vi "CalibrateSensors.vi"(5 "Static Load Cell":dbl) -> (1 "Static Load Cell Offset":string)   [LabVIEW 2018]
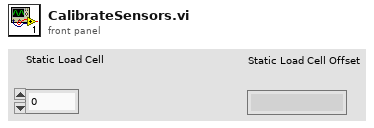
[diagram p1: front panel]
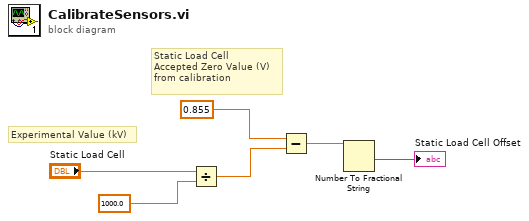
[diagram p0: block diagram]
diagram:
  # "Experimental Value (kV)"
  # "Static Load Cell\nAccepted Zero Value (V)\nfrom calibration"
  n1 = Divide(x="Static Load Cell", y=1000.0) -> (x/y=w2:dbl)
  n2 = Subtract(x=0.855, y=w2) -> (x-y=w1:dbl)
  n3 = Number To Fractional String(number=w1) -> (F-format string=→"Static Load Cell Offset":string)  [unwired: 3 in]
